vi "路径.vi"() -> ()   [LabVIEW 2023]
uses:
  <vilib>/Utility/sysdir.llb/System Directory Type.ctl
panel:
  in  "输入字符串":string
  in  "operation (0:open)":T1(ring)
  out "error out":errorcluster
  out "folder names":string[](array[string])
  out "filenames":string[](array[string])
  out "path out":path
  in  "system directory type":T2 items=["User Home"=0, "User Desktop"=1, "User Documents"=2, "User Application Data"=3, "User Preferences"=4, "User Temporary"=5, "Public Documents"=6, "Public Application Data"=7, "Public Preferences"=8, "Public Cache"=13, "System Core Libraries"=9, "System Installed Libraries"=10, "Application Files"=11, "Boot Volume Root"=12]
  out "current VI path":path
  # "路径"
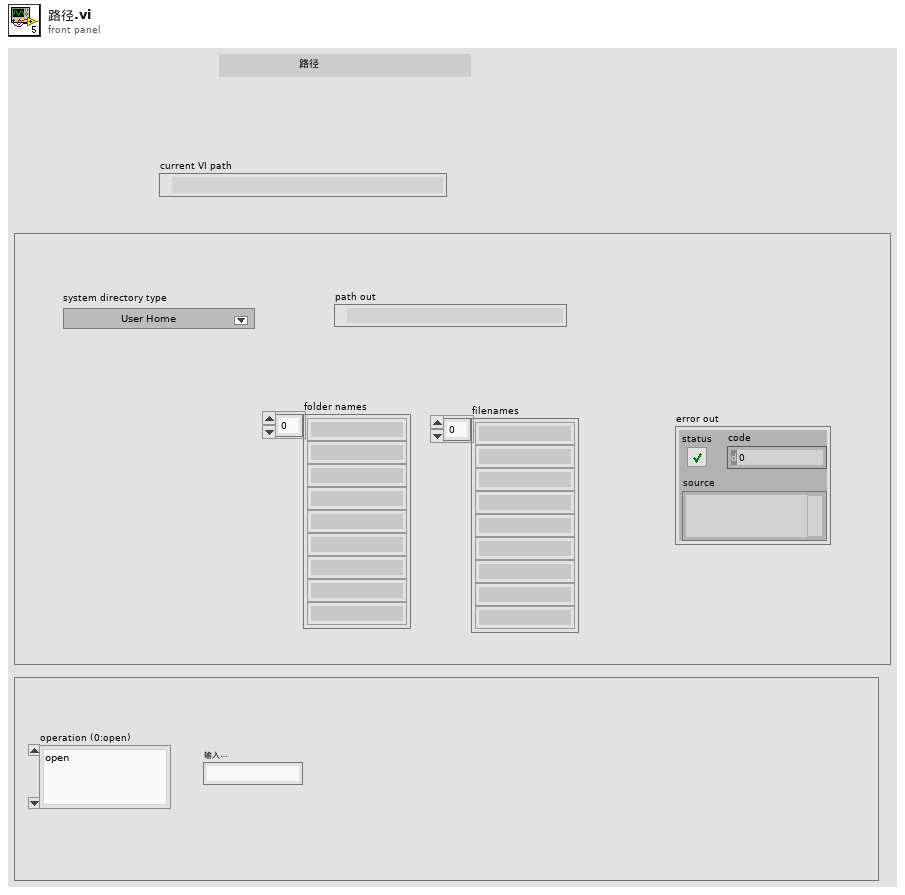
[diagram p1: front panel]
types:
  T1 = enum16{"open", "replace", "create", "open or create", "replace or create", "replace or create with confirmation"}
  T2 = typedef "System Directory Type.ctl" = i32
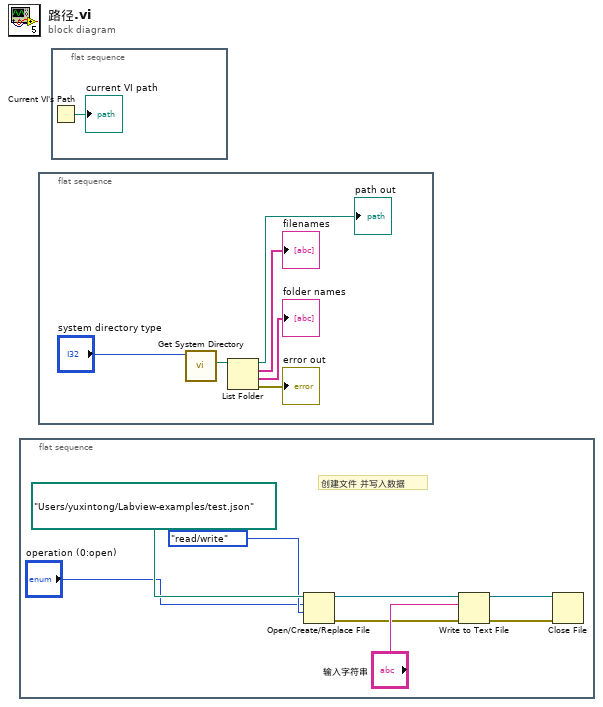
[diagram p0: block diagram]
diagram:
  n1 = flat-sequence {
    frame #0 {
      # "创建文件 并写入数据"
      n2 = Open/Create/Replace File(file path (use dialog)=path "/Users/yuxintong/Labview-examples/test.json", operation (0:open)="operation (0:open)", access (0:read/write)=enum16{"read/write", "read-only", "write-only"}."read/write") -> (refnum out=w5:refnum<file>, error out=w1:errorcluster)  [unwired: 3 in, 1 out]
      n3 = Write to Text File(file (use dialog)=w5, text="输入字符串", error in=w1) -> (refnum out=w3:refnum<file>, error out=w2:errorcluster)  [unwired: 1 in, 1 out]
      n4 = Close File(refnum=w3, error in=w2) -> ()  [unwired: 2 out]
    }
  }
  n5 = flat-sequence {
    frame #0 {
      n6 = call <vilib>:"Get System Directory.vi"("system directory type"="system directory type") -> ("system directory"=w13:path)  [unwired: 10 in]
      n7 = List Folder(path=w13) -> (path out=→"path out":path, filenames=→"filenames":string[], folder names=→"folder names":string[], error out=→"error out":errorcluster)  [unwired: 3 in]
    }
  }
  n8 = flat-sequence {
    frame #0 {
      n9 = Current VI's Path() -> (path=→"current VI path":path)
    }
  }
